vi "poly_notify_boolean_notifier_queue.vi"(2 "queue":refnum<queue>) -> (7 "notified?":bool)   [LabVIEW 2015]
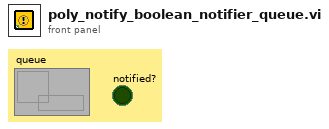
[diagram p1: front panel]
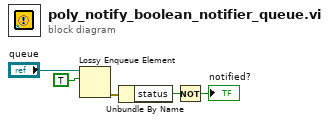
[diagram p0: block diagram]
diagram:
  n1 = Lossy Enqueue Element(queue="queue", element=TRUE) -> (error out=w2:errorcluster)  [unwired: 1 in, 3 out]
  n2 = Unbundle By Name(w2) -> ("status"=w5:bool)
  n3 = Not(x=w5) -> (.not. x?=→"notified?":bool)
